vi "GENERATEDUMMYIMAGE.vi"(1 "Numeric":i32, 2 "amplitude":dbl=1.0) -> (0 "Gaussian Monopulse":dbl[][](graph))   [LabVIEW 2011]
uses:
  NI_AALBase.lvlib
panel:
  out "x-y":u32
  out "min value":dbl
  out "max value":dbl
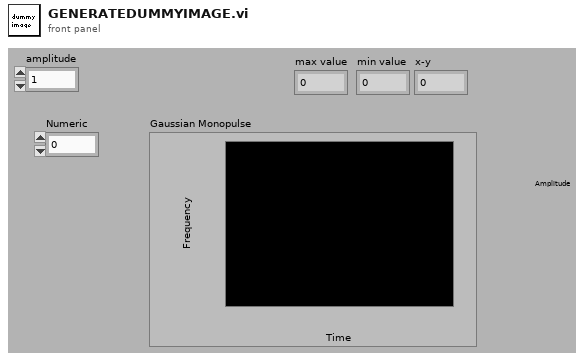
[diagram p1: front panel]
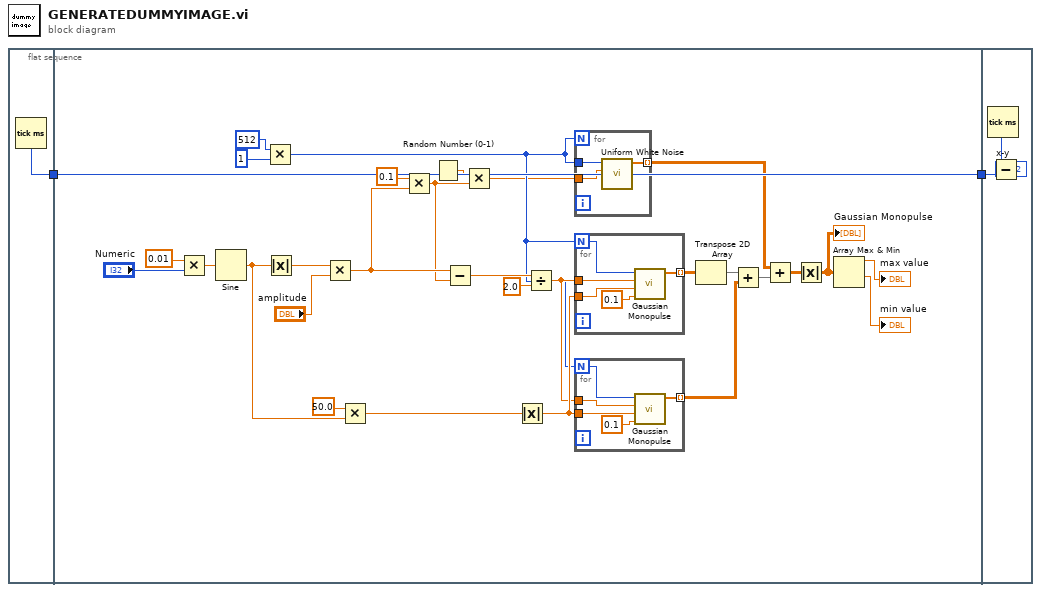
[diagram p0: block diagram]
diagram:
  n1 = flat-sequence {
    tunnel: [w3] -> w2
    tunnel: w2 -> [w16]
    tunnel: [w16] -> w1
    tunnel: w1 -> [w48]
    frame #0 {
      n2 = Tick Count (ms)() -> (millisecond timer value=w3:u32)
    }
    frame #1 {
      n3 = Multiply(x=0.01, y="Numeric") -> (x*y=w30:dbl)
      n4 = Sine(x=w30) -> (sin(x)=w25:dbl)
      n5 = Multiply(x=512, y=1) -> (x*y=w12:i32)
      n6 = Absolute Value(x=w25) -> (abs(x)=w23:dbl)
      n7 = Multiply(x=w23, y="amplitude") -> (x*y=w22:dbl)
      n8 = Multiply(x=50.0, y=w25) -> (x*y=w8:dbl)
      n9 = Multiply(x=0.1, y=w22) -> (x*y=w21:dbl)
      n10 = Random Number (0-1)() -> (number: 0 to 1=w10:dbl)
      n11 = Subtract(x=w22, y=w21) -> (x-y=w26:dbl)
      n12 = Multiply(x=w10, y=w21) -> (x*y=w9:dbl)
      n13 = Absolute Value(x=w8) -> (abs(x)=w31:dbl)
      n14 = Divide(x=w26, y=2.0) -> (x/y=w27:dbl)
      n15 = for {
        N: w12 -> [_]
        tunnel: [w36] -> w4 mode=indexing
        tunnel: w12 -> [w35]
        tunnel: w9 -> [w34]
        n16 = call "Uniform White Noise.vi"("amplitude"=w34, "samples"=w35) -> ("uniform white noise"=w36:dbl[])  [unwired: 8 in, 1 out]
      }
      n17 = for {
        N: w12 -> [w43]
        tunnel: w31 -> [w46]
        tunnel: [w44] -> w15 mode=indexing
        tunnel: w27 -> [w42]
        n18 = call "Gaussian Monopulse.vi"("delta t (s)"=0.1, "delay (s)"=w46, "amplitude"=w42, "samples"=w43) -> ("Gaussian Monopulse"=w44:dbl[])  [unwired: 6 in, 1 out]
      }
      n19 = for {
        N: w12 -> [w38]
        tunnel: w31 -> [w41]
        tunnel: [w39] -> w6 mode=indexing
        tunnel: w27 -> [w37]
        n20 = call "Gaussian Monopulse.vi"("delta t (s)"=0.1, "delay (s)"=w41, "amplitude"=w37, "samples"=w38) -> ("Gaussian Monopulse"=w39:dbl[])  [unwired: 6 in, 1 out]
      }
      n21 = Transpose 2D Array(2D array=w15) -> (transposed array=w32:dbl[][])
      n22 = Add(x=w32, y=w6) -> (x+y=w5:dbl[][])
      n23 = Add(x=w4, y=w5) -> (x+y=w18:dbl[][])
      n24 = Absolute Value(x=w18) -> (abs(x)=w17:dbl[][])
      "Gaussian Monopulse" <- w17
      n25 = Array Max & Min(array=w17) -> (max value=→"max value":dbl, min value=→"min value":dbl)  [unwired: 2 out]
    }
    frame #2 {
      n26 = Tick Count (ms)() -> (millisecond timer value=w49:u32)
      n27 = Subtract(x=w49, y=w48) -> (x-y=→"x-y":u32)
    }
  }
